vi "Count Status.vi"(10 "Status":T1, 11 "Method Result in":T2) -> (2 "Count":i32, 3 "Method Result out":T2)   [LabVIEW 2020, in "Method Result.lvlib"]
uses:
  Method Result.lvlib
  Method Result type.ctl
  Assertion Result/Public/TypeDefs/Status.ctl
  Assertion Result/Assertion Result type.ctl
  Assertion Result/Public/TypeDefs/Assertion Type.ctl
  Assertion Result/Assertion Result.lvlib
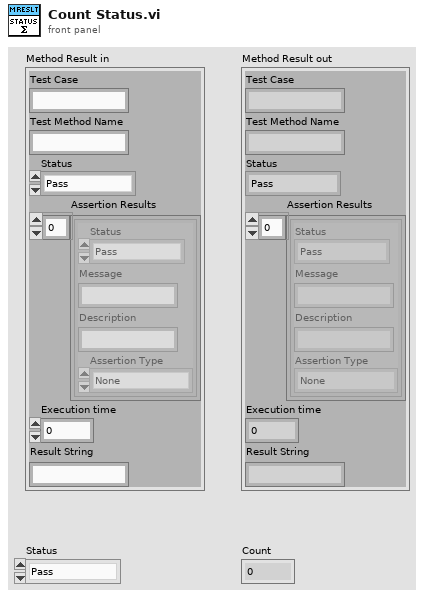
[diagram p1: front panel]
types:
  T1 = typedef "Assertion Result.lvlib/Status.ctl" = enum16{"Pass", "Fail", "Error", "Skipped", "Setup Error", "Broken", "Teardown Error"}
  T2 = typedef "Method Result.lvlib/Method Result type.ctl" = cluster{"Test Case":string, "Test Method Name":string, "Status":T1, "Assertion Results":T3[], "Execution time":dbl, "Result String":string}
  T3 = typedef "Assertion Result.lvlib/Assertion Result type.ctl" = cluster{"Status":T1, "Message":string, "Description":string, "Assertion Type":T4}
  T4 = typedef "Assertion Result.lvlib/Assertion Type.ctl" = enum16{"None", "Pass", "Fail", "Skip", "Pass if Equal", "Fail if Equal", "Pass if Error", "Fail if Error", "Pass if", "Fail if"}
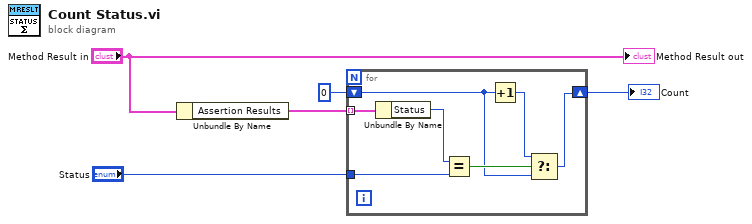
[diagram p0: block diagram]
diagram:
  n1 = Unbundle By Name("Method Result in") -> ("Assertion Results"=w4:T3[])
  n2 = for {
    tunnel: w4 -> [w12] mode=indexing
    shift-right: [w7] -> w3
    shift-left: 0 -> [w8]
    tunnel: "Status" -> [w6]
    n3 = Unbundle By Name(w12) -> ("Status"=w11:T1)
    n4 = Equal?(x=w11, y=w6) -> (x = y?=w10:bool)
    n5 = Increment(x=w8) -> (x+1=w9:i32)
    n6 = Select(t=w9, s=w10, f=w8) -> (s? t:f=w7:i32)
  }
  "Count" <- w3
  "Method Result out" <- "Method Result in"
